vi "Write RIO device.vi"(8 "error in (no error)":errorcluster, 10 "RIO device":string, 11 "PL_Target Runtime in":refnum<class "PL_Target Runtime.lvclass">) -> (0 "error out":errorcluster, 3 "PL_Target Runtime out":refnum<class "PL_Target Runtime.lvclass">)   [LabVIEW 2013, in "PL_Target Runtime.lvclass"]
uses:
  PL_Target Runtime.lvclass
  PL_Target Runtime.lvclass/PL_Target Runtime.ctl
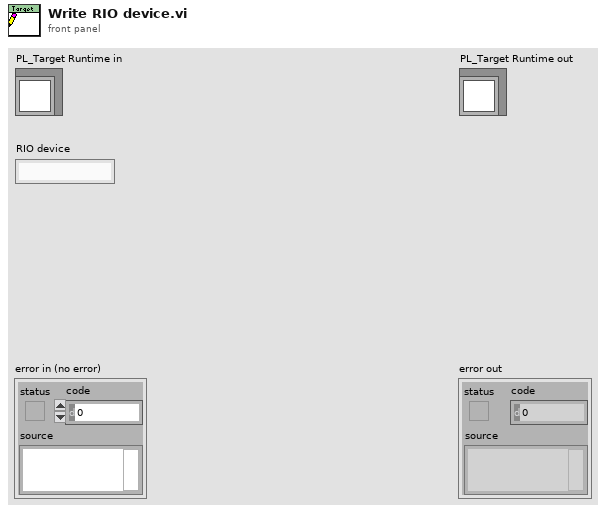
[diagram p1: front panel]
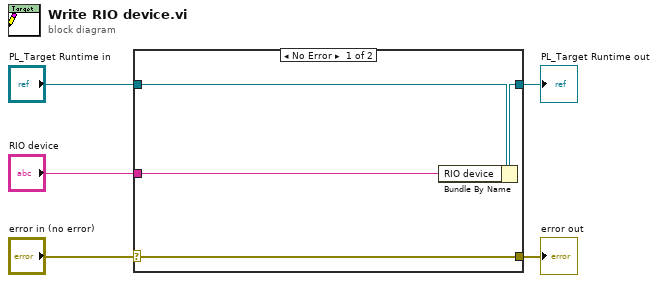
[diagram p0: block diagram]
diagram:
  n1 = case shown="No Error" "error in (no error)" {
    selector: "error in (no error)" -> [w9 w10]
    tunnel: [w9 w10] -> w4
    tunnel: [w7 w11] -> w2
    tunnel: "PL_Target Runtime in" -> [w8 w11]
    tunnel: "RIO device" -> [w6 _]
    frame No Error {
      n2 = Bundle By Name(cluster=w8, "RIO device"=w6) -> (w7:refnum<class "PL_Target Runtime.lvclass">)
    }
    frame Error {
    }
  }
  "error out" <- w4
  "PL_Target Runtime out" <- w2
